vi "LabVLC - StopControl.vi"(2 "error in (no error)":errorcluster, 3 "struct":T1={"media_ptr"=0, "vlc_inst_ptr"=0, "path in"=path "C:/Program Files (x86)/VideoLAN/VLC/libvlc.dll"}) -> (0 "error out":errorcluster, 1 "out":T1)   [LabVIEW 2014]
doc: "Stop VLC playback. Pass in the VLC instance handle created in the initialization for an error-free close. Also accepts the media pointer."
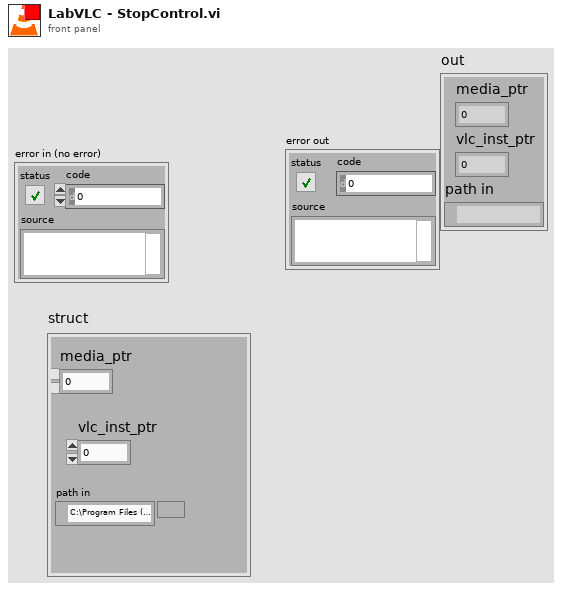
[diagram p1: front panel]
types:
  T1 = cluster{"media_ptr":i32, "vlc_inst_ptr":i32, "path in":path}
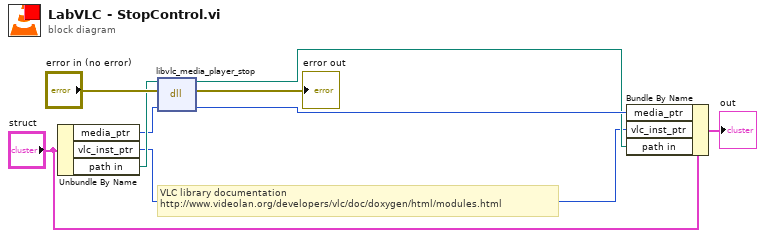
[diagram p0: block diagram]
diagram:
  # "VLC library documentation\nhttp://www.videolan.org/developers/vlc/doc/doxygen/html/modules.html"
  n1 = Unbundle By Name("struct") -> ("media_ptr"=w5:i32, "vlc_inst_ptr"=w2:i32, "path in"=w6:path)
  n2 = dll-call lib="C:/Program Files (x86)/VideoLAN/VLC/libvlc.dll" fn="libvlc_media_player_stop"(path in=w6, error in="error in (no error)", "media_pointer"=w5) -> (path out=w3:path, error out=→"error out":errorcluster, "media_pointer"=w4:i32)  [unwired: 2 in]
  n3 = Bundle By Name(cluster="struct", "media_ptr"=w4, "vlc_inst_ptr"=w2, "path in"=w3) -> (→"out":T1)
